vi "Read Loop Period in ms (10).vi"(8 "error in (no error)":errorcluster, 11 "Analog Reader Helper in":refnum<class "Analog Reader Helper.lvclass">) -> (0 "error out":errorcluster, 2 "Loop Period in ms (10)":u32=10, 3 "Analog Reader Helper out":refnum<class "Analog Reader Helper.lvclass">)   [LabVIEW 2024]
uses:
  Analog Reader Helper.lvclass
  Analog Reader Helper.lvclass/Analog Reader Helper.ctl
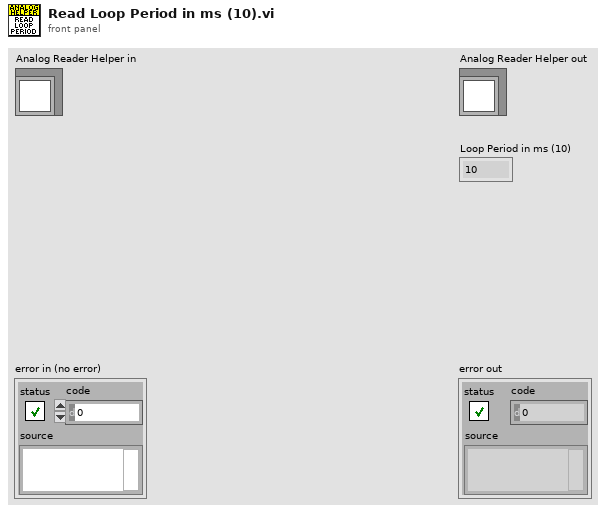
[diagram p1: front panel]
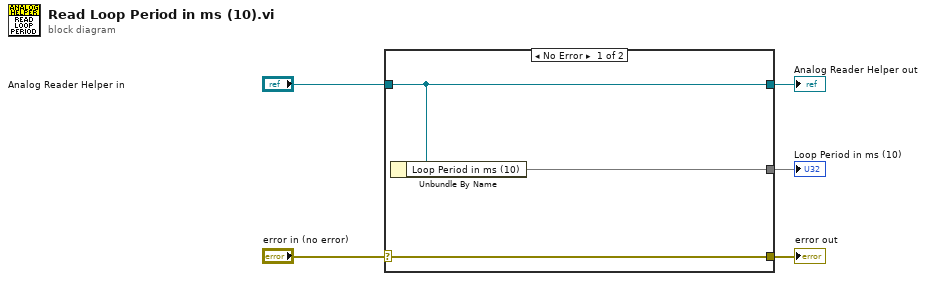
[diagram p0: block diagram]
diagram:
  n1 = case shown="No Error" "error in (no error)" {
    selector: "error in (no error)" -> [w8 w9]
    tunnel: [w8 w9] -> w4
    tunnel: [w7 w10] -> w2
    tunnel: "Analog Reader Helper in" -> [w7 w10]
    tunnel: [w6 _] -> w1
    frame No Error {
      n2 = Unbundle By Name(w7) -> ("Loop Period in ms (10)"=w6)
    }
    frame Error {
    }
  }
  "error out" <- w4
  "Analog Reader Helper out" <- w2
  "Loop Period in ms (10)" <- w1
